vi "Error Handler.vi"(8 "error in (no error)":errorcluster, 11 "Measurements in":refnum<class "Measurement.lvclass">) -> (0 "error out":errorcluster, 2 "Cancel tests":bool, 3 "Measurements out":refnum<class "Measurement.lvclass">)   [LabVIEW 2020, in "Measurement.lvclass"]
doc: "Error handler for the test.\nOnly override if special error handling is needed"
uses:
  Measurement.lvclass
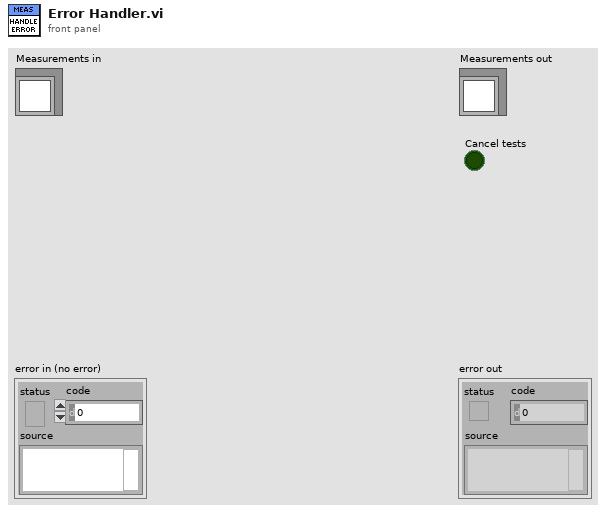
[diagram p1: front panel]
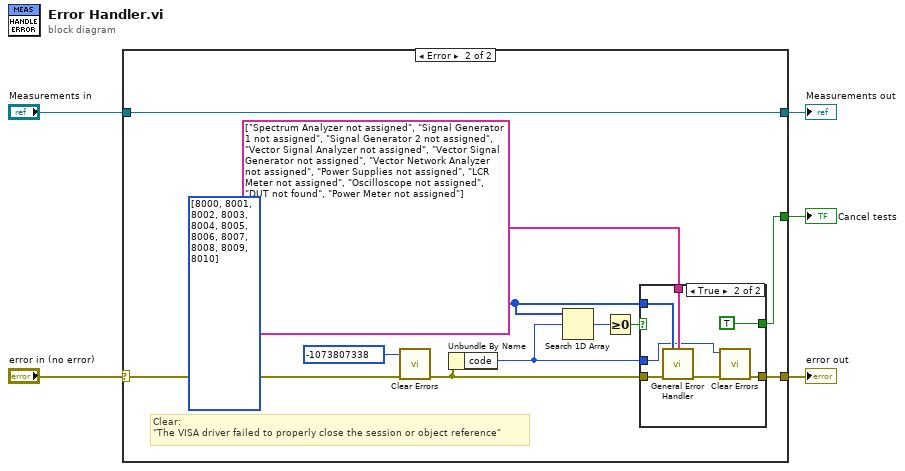
[diagram p0: block diagram]
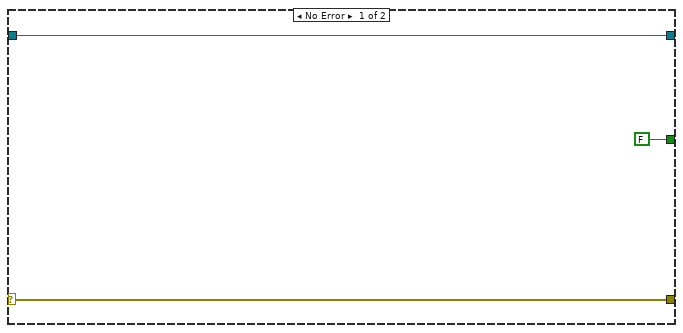
[diagram p2: hidden frame]
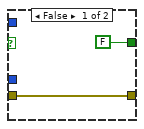
[diagram p3: hidden frame]
diagram:
  n1 = case shown="Error" "error in (no error)" {
    selector: "error in (no error)" -> [w7 w13]
    tunnel: [w7 w16] -> w4
    tunnel: [w8 w19] -> w2
    tunnel: "Measurements in" -> [w8 w19]
    tunnel: [FALSE w15] -> w1
    frame No Error {
    }
    frame Error {
      w12 = i32[] [8000, 8001, 8002, 8003, 8004, 8005, 8006, 8007, 8008, 8009, 8010] ("[user-defined codes]")
      # "Clear:\n\"The VISA driver failed to properly close the session or object reference\""
      n2 = call <vilib>:"Clear Errors.vi"("error in (no error)"=w13, "specific error code to clear (0: all)"=-1073807338) -> ("error out"=w10:errorcluster)  [unwired: 4 in, 1 out]
      n3 = Unbundle By Name(w10) -> ("code"=w9:i32)
      n4 = Search 1D Array(1D array=w12, element=w9) -> (index of element=w18:i32)  [unwired: 1 in]
      n5 = Greater Or Equal To 0?(x=w18) -> (x >= 0?=w17:bool)
      n6 = case shown="True" w17 {
        tunnel: [w20 w28] -> w16
        tunnel: [FALSE TRUE] -> w15
        tunnel: w12 -> [_ w26]
        tunnel: string[] ["Spectrum Analyzer not assigned", "Signal Generator 1 not assigned", "Signal Generator 2 not assigned", "Vector Signal Analyzer not assigned", "Vector Signal Generator not assigned", "Vector Network Analyzer not assigned", "Power Supplies not assigned", "LCR Meter not assigned", "Oscilloscope not assigned", "DUT not found", "Power Meter not assigned"] ("[user-defined descriptions]") -> [_ w25]
        tunnel: w10 -> [w20 w24]
        tunnel: w9 -> [_ w22]
        frame False {
        }
        frame True {
          n7 = call <vilib>:"General Error Handler.vi"("[user-defined codes]"=w26, "[user-defined descriptions]"=w25, "error in (no error)"=w24) -> ("error out"=w23:errorcluster)  [unwired: 8 in, 4 out]
          n8 = call <vilib>:"Clear Errors.vi"("error in (no error)"=w23, "specific error code to clear (0: all)"=w22) -> ("error out"=w28:errorcluster)  [unwired: 4 in, 1 out]
        }
      }
    }
  }
  "error out" <- w4
  "Measurements out" <- w2
  "Cancel tests" <- w1
